vi "createPIDParametersFrame.vi"(0 "FAILC in":refnum<class "FAILC.lvclass">, 1 "WaitForTrigger":bool, 2 "TriggerIRQ":bool, 3 "PIDNumber":u8, 4 "FAPID":T1, 5 "error in (no error)":errorcluster) -> (14 "FAILC out":refnum<class "FAILC.lvclass">, 15 "Frame":T2 {"Data" format="%02x"}, 19 "error out":errorcluster)   [LabVIEW 2015, in "RTFAILC.lvlib" / "FAILC.lvclass"]
uses:
  FAILC.lvclass
  Common_RT_Modbus/DataTypes/Frame.ctl
  DataTypes/FAPID.ctl
  Common_RT_Modbus/DynamicFrameBuilder/DynamicFrameBuilder.lvclass
  Common_RT_ILC/ILC/ILC.lvclass/ILC.ctl
  Common_RT_ILC/ILC/ILC.lvclass
  Common_RT_Modbus/RTModbus.lvlib
  RTFAILC.lvlib
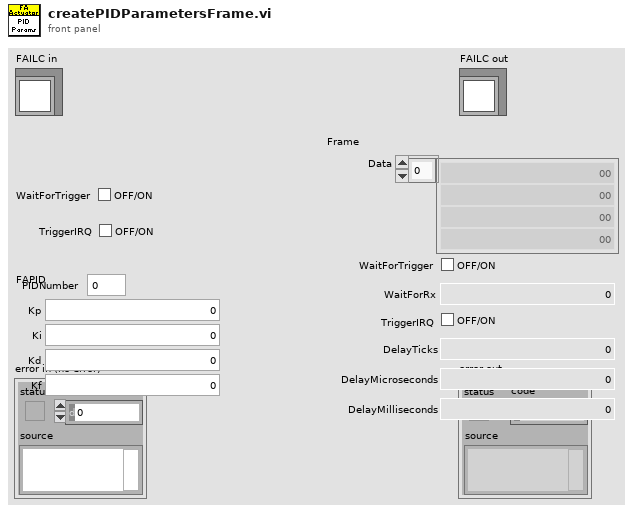
[diagram p1: front panel]
types:
  T1 = typedef "RTFAILC.lvlib/FAPID.ctl" = cluster{"Kp":sgl, "Ki":sgl, "Kd":sgl, "Kf":sgl}
  T2 = typedef "RTModbus.lvlib/Frame.ctl" = cluster{"Data":u8[], "WaitForTrigger":bool, "WaitForRx":u16, "TriggerIRQ":bool, "DelayTicks":u16, "DelayMicroseconds":u16, "DelayMilliseconds":u16}
  T3 = typedef "RTILC.lvlib/ILCData.ctl" = cluster{"Constants":T4, "Command":T5, "Telemetry":T7, "Responses":T8}
  T4 = typedef "RTILC.lvlib/ILCConstants.ctl" = cluster{"Subnet":u8, "Address":u8}
  T5 = typedef "RTILC.lvlib/ILCCommand.ctl" = cluster{"ILCMode":u16, "TemporaryAddress":u8, "ADCScanRate":T6, "ADCChannel":u8, "ADCOffset":sgl, "ADCSensitivity":sgl}
  T6 = typedef "RTILC.lvlib/ILCScanRates.ctl" = u8
  T7 = typedef "RTILC.lvlib/ILCTelemetry.ctl" = cluster{"UniqueID":u64, "FirmwareType":u8, "NetworkNodeType":u8, "ILCOption":u8, "NetworkNodeOption":u8, "MajorRevision":u8, "MinorRevision":u8, "FirmwareName":string, "ILCMode":u16, "MajorFault":bool, "MinorFault":bool, "FaultOverride":bool, "UniqueIDCRCMismatch":bool, "AppTypeNodeTypeMismatch":bool, "AppMissing":bool, "AppCRCMismatch":bool, "TEDSNotFound":bool, "TEDS1Mismatch":bool, "TEDS2Mismatch":bool, "WatchdogResetDetected":bool, "BrownoutDetected":bool, "EventTrapResetDetected":bool, "TemporaryAddress":u8, "ADCScanRate":T6, "DAC1":u16, "DAC2":u16, "DAC3":u16, "DAC4":u16, "MainADCCalibrationK":sgl[], "MainSensorOffset":sgl[], "MainSensorSensitivity":sgl[], "BackupADCCalibrationK":sgl[], "BackupSensorOffset":sgl[], "BackupSensorSensitivity":sgl[]}
  T8 = typedef "RTILC.lvlib/ILCResponses.ctl" = cluster{"ReportServerID":T9, "ReportServerStatus":T9, "ILCMode":T9, "SetTemporaryAddress":T9, "Reset":T9, "ADCScanRate":T9, "ADCOffsetSensitivity":T9, "ReadDAC":T9, "ReadCalibration":T9}
  T9 = typedef "RTModbus.lvlib/ExceptionCodes.ctl" = u16
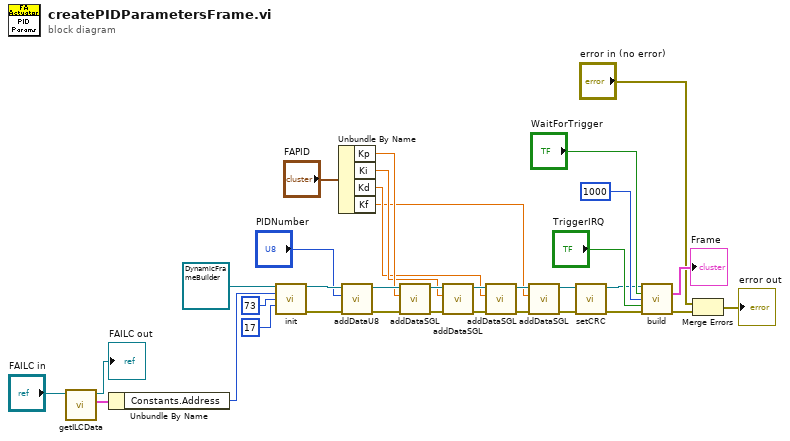
[diagram p0: block diagram]
diagram:
  n1 = call "getILCData.vi"("ILC in"="FAILC in") -> ("ILCData"=w32:T3, "ILC out"=→"FAILC out":refnum<class "FAILC.lvclass">)  [unwired: 9 in]
  n2 = Unbundle By Name(w32) -> ("Constants.Address"=w31:u8)
  n3 = call "init.vi"("DynamicFrameBuilder in"=refnum<class "DynamicFrameBuilder.lvclass"> refnum ("RTModbus.lvlib:DynamicFrameBuilder.lvclass"), "Address"=w31, "Function"=u8 73, "DataSize"=17) -> ("DynamicFrameBuilder out"=w11:refnum<class "DynamicFrameBuilder.lvclass">, "error out"=w28:errorcluster)  [unwired: 10 in]
  n4 = Unbundle By Name("FAPID") -> ("Kp"=w8:sgl, "Ki"=w7:sgl, "Kd"=w6:sgl, "Kf"=w5:sgl)
  n5 = call "addDataU8.vi"("error in (no error)"=w28, "Data"="PIDNumber", "DynamicFrameBuilder in"=w11) -> ("error out"=w27:errorcluster, "DynamicFrameBuilder out"=w12:refnum<class "DynamicFrameBuilder.lvclass">)  [unwired: 7 in]
  n6 = call "addDataSGL.vi"("error in (no error)"=w27, "Data"=w8, "DynamicFrameBuilder in"=w12) -> ("error out"=w26:errorcluster, "DynamicFrameBuilder out"=w13:refnum<class "DynamicFrameBuilder.lvclass">)  [unwired: 7 in]
  n7 = call "addDataSGL.vi"("error in (no error)"=w26, "Data"=w7, "DynamicFrameBuilder in"=w13) -> ("error out"=w25:errorcluster, "DynamicFrameBuilder out"=w14:refnum<class "DynamicFrameBuilder.lvclass">)  [unwired: 7 in]
  n8 = call "addDataSGL.vi"("error in (no error)"=w25, "Data"=w6, "DynamicFrameBuilder in"=w14) -> ("error out"=w24:errorcluster, "DynamicFrameBuilder out"=w15:refnum<class "DynamicFrameBuilder.lvclass">)  [unwired: 7 in]
  n9 = call "addDataSGL.vi"("error in (no error)"=w24, "Data"=w5, "DynamicFrameBuilder in"=w15) -> ("error out"=w23:errorcluster, "DynamicFrameBuilder out"=w16:refnum<class "DynamicFrameBuilder.lvclass">)  [unwired: 7 in]
  n10 = call "setCRC.vi"("error in (no error)"=w23, "DynamicFrameBuilder in"=w16) -> ("error out"=w22:errorcluster, "DynamicFrameBuilder out"=w17:refnum<class "DynamicFrameBuilder.lvclass">)  [unwired: 8 in]
  n11 = call "build.vi"("DynamicFrameBuilder in"=w17, "WaitForTrigger"="WaitForTrigger", "WaitForRxTimeout"=u16 1000, "TriggerIRQ"="TriggerIRQ", "error in (no error)"=w22) -> ("Frame"=→"Frame":T2, "error out"=w3:errorcluster)  [unwired: 8 in, 1 out]
  n12 = Merge Errors("error in (no error)", w3) -> (→"error out":errorcluster)
